vi "helper-wind-status.vi"(11 "Ndir":T1=enum."NE") -> (3 "Value":string)   [LabVIEW 2024]
uses:
  controls/wind-directions.ctl
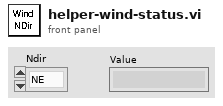
[diagram p1: front panel]
types:
  T1 = typedef "wind-directions.ctl" = enum16{"N", "NE", "E", "SE", "S", "SW", "W", "NW"}
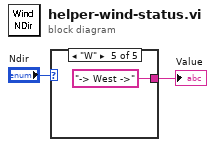
[diagram p0: block diagram]
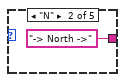
[diagram p3: hidden frame]
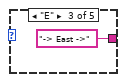
[diagram p4: hidden frame]
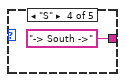
[diagram p5: hidden frame]
diagram:
  n1 = case shown="\"W\"" "Ndir" {
    tunnel: [_ "-> North ->" ("Value") "-> East ->" ("Value") "-> South ->" ("Value") "-> West ->" ("Value")] -> w1
    frame Default {
    }
    frame "N" {
    }
    frame "E" {
    }
    frame "S" {
    }
    frame "W" {
    }
  }
  "Value" <- w1
